vi "Generate Digital Sine Wave.vi"(5 "Command_Data array":i16[](array[numeric]), 6 "Number of Bits":u32=16, 7 "Full scale range":dbl=5.0 format="%#_13g", 9 "Amplitude stop":dbl=4.5 format="%#_13g", 10 "Amplitude start":dbl=0.5 format="%#_13g", 11 "Frequency":dbl=100.0 format="%#_13g") -> (1 "Points per cycle":i32, 3 "Digital Sine waveform":i16[](graph))   [LabVIEW 2021]
uses:
  <vilib>/measure/NI_MABase.lvlib
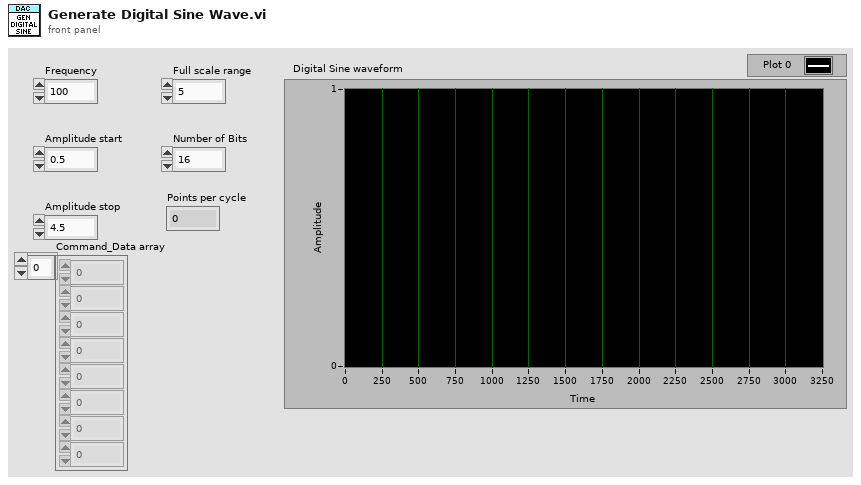
[diagram p1: front panel]
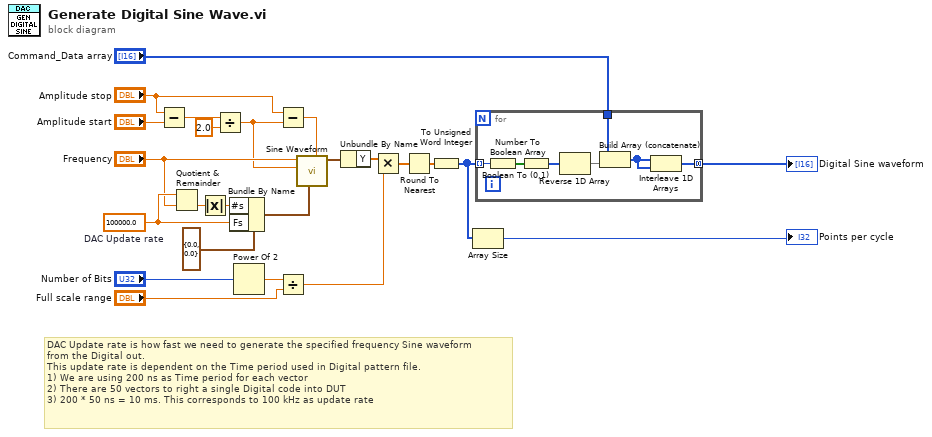
[diagram p0: block diagram]
diagram:
  w19 = 100000.0  # DAC Update rate
  # "DAC Update rate is how fast we need to generate the specified frequency Sine waveform\nfrom the Digital out.\nThis update rate is dependent on the Time period used in Digital pattern file.\n1) We are using 200 ns as Time period for each vector\n2) There are 50 vectors to right a single Digital code into DUT\n3) 200 * 50 ns = 10 ms. This corresponds to 100 kHz as update rate"
  n1 = Subtract(x="Amplitude stop", y="Amplitude start") -> (x-y=w11:dbl)
  n2 = Quotient & Remainder(x=w19, y="Frequency") -> (floor(x/y)=w17:dbl)  [unwired: 1 out]
  n3 = Absolute Value(x=w17) -> (abs(x)=w16:dbl)
  n4 = Divide(x=w11, y=2.0) -> (x/y=w10:dbl)
  n5 = Bundle By Name(cluster=cluster{"Fs":dbl, "#s":dbl} {"Fs"=0.0, "#s"=0.0} ("sampling info"), "#s"=w16, "Fs"=w19) -> (w15:cluster{"Fs":dbl, "#s":dbl})
  n6 = Power Of 2(x="Number of Bits") -> (2^x=w6:dbl)
  n7 = Subtract(x="Amplitude stop", y=w10) -> (x-y=w8:dbl)
  n8 = Divide(x=w6, y="Full scale range") -> (x/y=w5:dbl)
  n9 = call <vilib>:"Sine Waveform.vi"("offset"=w8, "sampling info"=w15, "amplitude"=w10, "frequency"="Frequency") -> ("signal out"=w24:waveform(dbl))  [unwired: 6 in, 1 out]
  n10 = Unbundle By Name(w24) -> ("Y"=w13:dbl[])
  n11 = Multiply(x=w13, y=w5) -> (x*y=w23:dbl[])
  n12 = Round To Nearest(number=w23) -> (nearest integer value=w22:dbl[])
  n13 = To Unsigned Word Integer(number=w22) -> (unsigned 16bit integer=w3:u16[])
  n14 = Array Size(array=w3) -> (size(s)=→"Points per cycle":i32)
  n15 = for {
    tunnel: [w29] -> w4 mode=concatenating
    tunnel: w3 -> [w28] mode=indexing
    tunnel: "Command_Data array" -> [w26]
    n16 = Number To Boolean Array(number=w28) -> (Boolean array=w31:bool[])
    n17 = Boolean To (0,1)(Boolean=w31) -> (0, 1=w30:i16[])
    n18 = Reverse 1D Array(array=w30) -> (reversed array=w27:i16[])
    n19 = Build Array (concatenate)(w26, w27) -> (w25:i16[])
    n20 = Interleave 1D Arrays(w25, w25) -> (w29:i16[])
  }
  "Digital Sine waveform" <- w4
